vi "CD Read Engine_Simulate Records_Create Activity Field.vi"(11 "activity flags":T1 {"bus" items=["BUSA", "BUSB", "BUSNONE"]}) -> (3 "Activity":u16 format="%.0x")   [LabVIEW 2017, in "Ballard MIL-1553 Engine.lvlib"]
uses:
  Ballard MIL-1553 Engine.lvlib
  <instrlib>/BTI1553Lib/Public/Controls/1553 Activity Flags.ctl
  <instrlib>/BTI1553Lib/BTI1553LV.lvlib
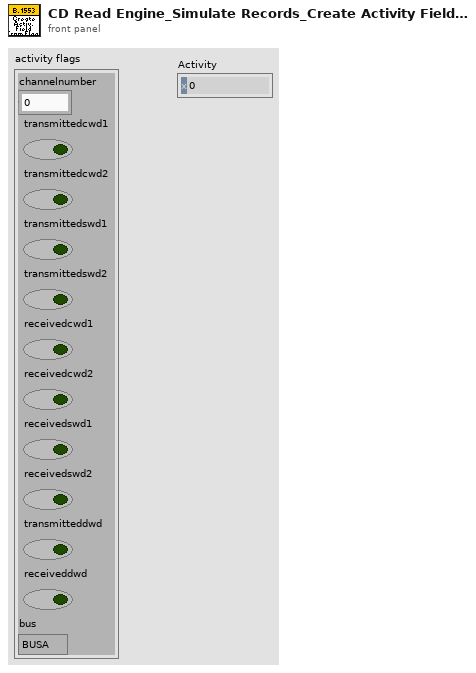
[diagram p1: front panel]
types:
  T1 = typedef "BTI1553LV.lvlib/1553 Activity Flags.ctl" = cluster{"channelnumber":i32, "transmittedcwd1":bool, "transmittedcwd2":bool, "transmittedswd1":bool, "transmittedswd2":bool, "receivedcwd1":bool, "receivedcwd2":bool, "receivedswd1":bool, "receivedswd2":bool, "transmitteddwd":bool, "receiveddwd":bool, "reserved1":i8, "reserved2":i8, "bus":u32}
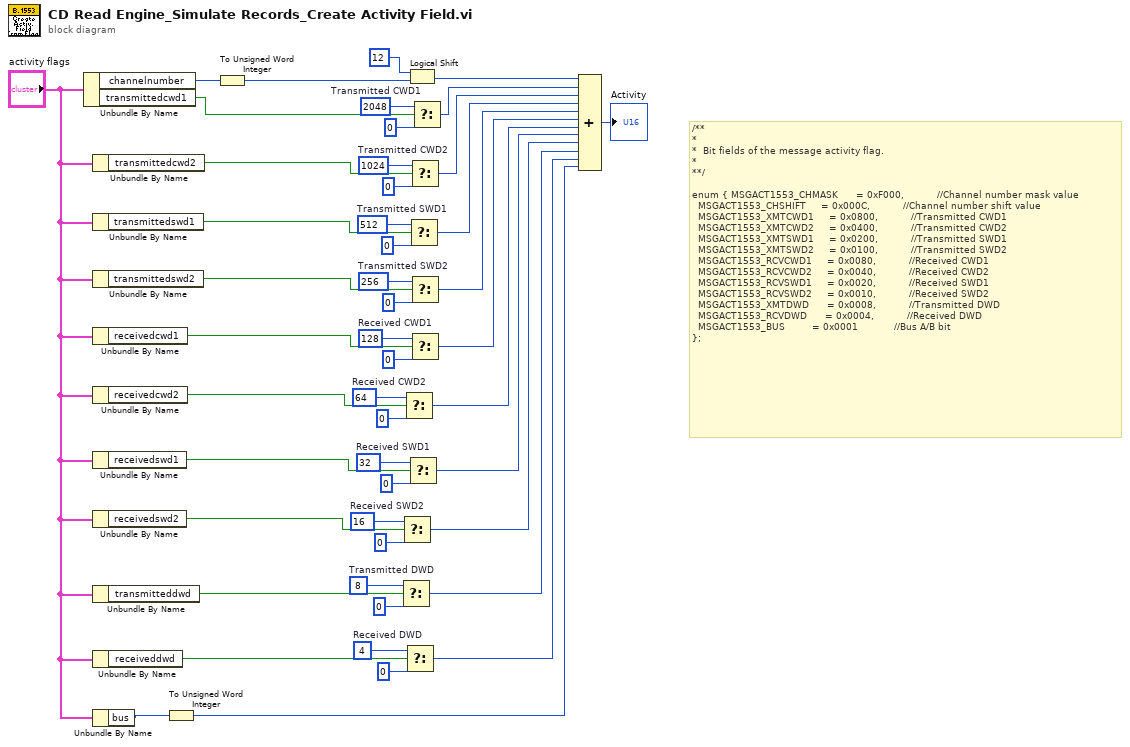
[diagram p0: block diagram]
diagram:
  w13 = u16 4  # Received DWD
  w10 = u16 8  # Transmitted DWD
  w19 = u16 16  # Received SWD2
  w16 = u16 32  # Received SWD1
  w23 = u16 64  # Received CWD2
  w27 = u16 128  # Received CWD1
  w31 = u16 256  # Transmitted SWD2
  w35 = u16 512  # Transmitted SWD1
  w39 = u16 1024  # Transmitted CWD2
  w45 = u16 2048  # Transmitted CWD1
  # "/**\n*\n*  Bit fields of the message activity flag.\n*\n**/\n\nenum {\tMSGACT1553_CHMASK      = 0xF000,           //Channel number mask value\n\t\tMSGACT1553_CHSHIFT     = 0x000C,           //Channel number shift value\n\t\tMSGACT1553_XMTCWD1     = 0x0800,           //Transmitted CWD1\n\t\tMSGACT1553_XMTCWD2     = 0x0400,           //Transmitted CWD2\n\t\tMSGACT1553_XMTSWD1     = 0x0200,           //Transmitted SWD1\n\t\tMSGACT1553_XMTSWD2     = 0x0100,           //Transmitted SWD2\n\t\tMSGACT1553_RCVCWD1     = 0x0080,           //Received CWD1\n\t\tMSGACT1553_RCVCWD2     = 0x0040,           //Received CWD2\n\t\tMSGACT1553_RCVSWD1     = 0x0020,           //Received SWD1\n\t\tMSGACT1553_RCVSWD2     = 0x0010,           //Received SWD2\n\t\tMSGACT1553_XMTDWD      = 0x0008,           //Transmitted DWD\n\t\tMSGACT1553_RCVDWD      = 0x0004,           //Received DWD\n\t\tMSGACT1553_BUS         = 0x0001            //Bus A/B bit\n};"
  n1 = Unbundle By Name("activity flags") -> ("channelnumber"=w48:i32, "transmittedcwd1"=w44:bool)
  n2 = Unbundle By Name("activity flags") -> ("transmittedcwd2"=w38:bool)
  n3 = Unbundle By Name("activity flags") -> ("transmittedswd1"=w36:bool)
  n4 = Unbundle By Name("activity flags") -> ("transmittedswd2"=w30:bool)
  n5 = Unbundle By Name("activity flags") -> ("receivedcwd1"=w28:bool)
  n6 = Unbundle By Name("activity flags") -> ("receivedcwd2"=w22:bool)
  n7 = Unbundle By Name("activity flags") -> ("receivedswd1"=w15:bool)
  n8 = Unbundle By Name("activity flags") -> ("receivedswd2"=w20:bool)
  n9 = Unbundle By Name("activity flags") -> ("transmitteddwd"=w11:bool)
  n10 = Unbundle By Name("activity flags") -> ("receiveddwd"=w14:bool)
  n11 = Unbundle By Name("activity flags") -> ("bus"=w3:u32)
  n12 = To Unsigned Word Integer(number=w3) -> (unsigned 16bit integer=w2:u16)
  n13 = To Unsigned Word Integer(number=w48) -> (unsigned 16bit integer=w41:u16)
  n14 = Select(t=w10, s=w11, f=u16 0) -> (s? t:f=w5:u16)
  n15 = Select(t=w19, s=w20, f=u16 0) -> (s? t:f=w6:u16)
  n16 = Select(t=w23, s=w22, f=u16 0) -> (s? t:f=w21:u16)
  n17 = Select(t=w13, s=w14, f=u16 0) -> (s? t:f=w4:u16)
  n18 = Logical Shift(y=i16 12, x=w41) -> (x << y=w46:u16)
  n19 = Select(t=w16, s=w15, f=u16 0) -> (s? t:f=w7:u16)
  n20 = Select(t=w35, s=w36, f=u16 0) -> (s? t:f=w33:u16)
  n21 = Select(t=w39, s=w38, f=u16 0) -> (s? t:f=w37:u16)
  n22 = Select(t=w31, s=w30, f=u16 0) -> (s? t:f=w29:u16)
  n23 = Select(t=w27, s=w28, f=u16 0) -> (s? t:f=w25:u16)
  n24 = Select(t=w45, s=w44, f=u16 0) -> (s? t:f=w42:u16)
  n25 = Compound Arithmetic op=ADD(w46, w42, w37, w33, w29, w25, w21, w7, w6, w5, w4, w2) -> (→"Activity":u16)
